vi "Fin_main.vi"(8 "Error In":errorcluster, 11 "Fin Arrangement (SORTED)":u8[](array[numeric])) -> (0 "Error Out":errorcluster)   [LabVIEW 2013]
uses:
  <vilib>/Platform/TimedLoop/XDataNode/timing_clust.ctl
  <vilib>/Platform/TimedLoop/XDataNode/nitl_modes.ctl
  <vilib>/Platform/TimedLoop/XDataNode/wakeup.ctl
  My Computer/Controls/Steering Mode.ctl
  My Computer/Controls/Fin Status.ctl
  <vilib>/platform/TimedLoop/XDataNode/XDataNode.xnode
  <vilib>/Platform/TimedLoop/XDataNode/XDNodeRunTimeDep.lvlib
panel:
  out "x-y":dbl
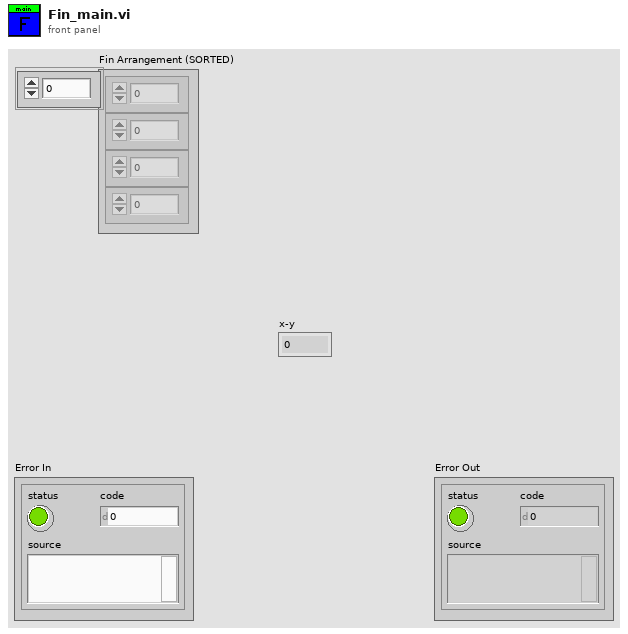
[diagram p1: front panel]
types:
  T1 = typedef "XDNodeRunTimeDep.lvlib/timing_clust.ctl" = cluster{"Expected End [f-1]":u64, "Actual End [f-1]":u64, "Finished Late? [f-1]":bool, "Expected End [i-1]":u64, "Actual End [i-1]":u64, "Finished Late? [i-1]":bool, "Expected Start [i]":u64, "Actual Start [i]":u64, "Expected Start [f]":u64, "Actual Start [f]":u64, "Source Name":string, "Structure Name":string, "Period":i64, "Deadline":i64, "Offset":i64, "Start":i64, "Priority":i32, "Timeout":i32, "Mode":T2, "Wakeup Reason":T3, "Error":errorcluster, "Source Type":string, "Secondary Source Type":string, "Global End Time":u64, "Global Start Time":u64, "Frame Duration":u64, "Iteration Duration":u64, "Assigned CPU":i32, "I/O Scan Engine Mode":u32}
  T2 = typedef "XDNodeRunTimeDep.lvlib/nitl_modes.ctl" = enum32{"No Change", "Process missed periods, maintain original phase", "Discard missed periods, maintain original phase", "Process missed periods, ignore original phase", "Discard missed periods, ignore original phase"}
  T3 = typedef "XDNodeRunTimeDep.lvlib/wakeup.ctl" = enum32{"Normal", "Aborted", "Asynchronous wakeup", "Timing source error", "Timed loop error", "Timeout"}
  T4 = typedef "Steering Mode.ctl" = enum16{"Intuitive Steering", "Control Allocation", "Individually"}
  T5 = typedef "Servo Position.ctl" = dbl[][]
  T6 = typedef "Fin Status.ctl" = u32[]
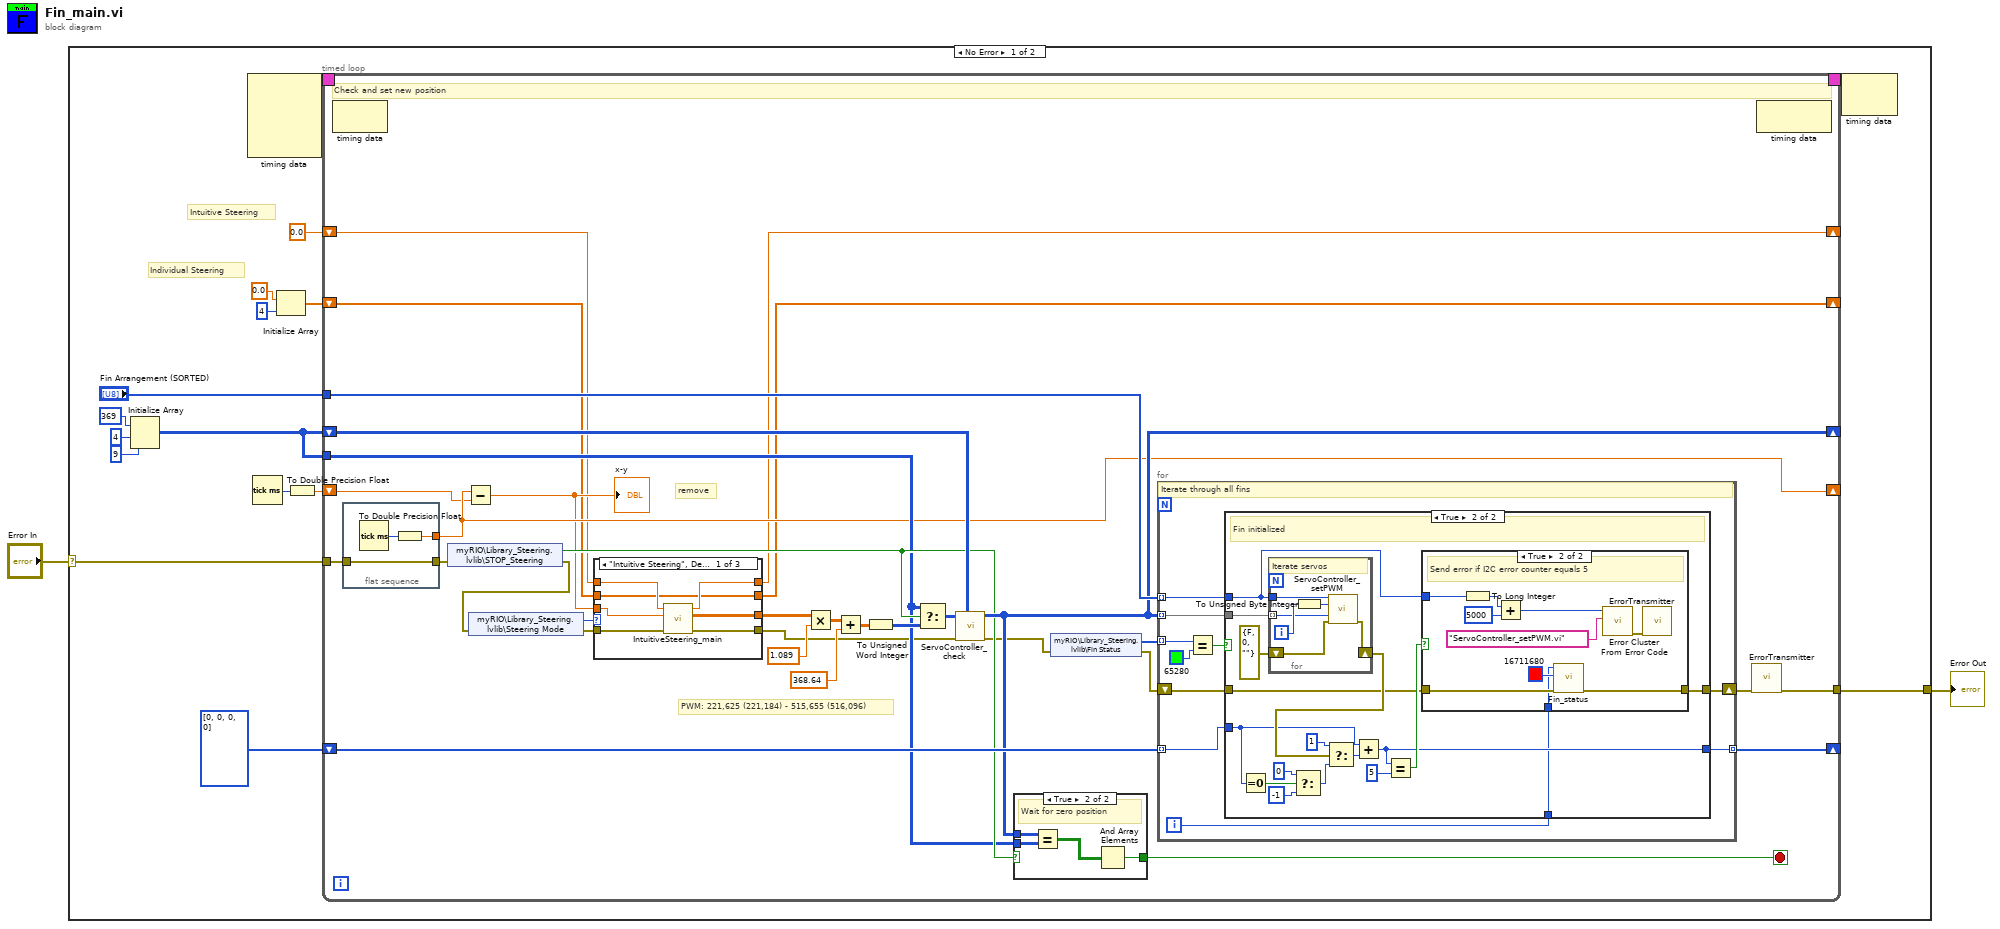
[diagram p0: block diagram]
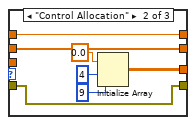
[diagram p2: hidden frame]
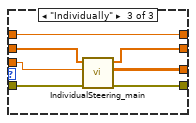
[diagram p3: hidden frame]
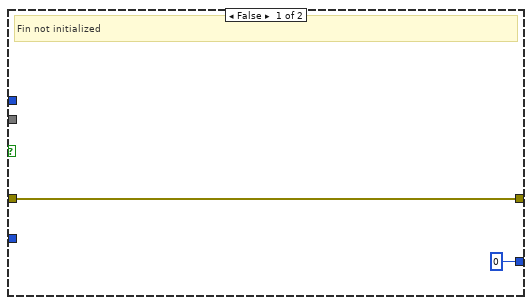
[diagram p5: hidden frame]
diagram:
  n1 = case shown="No Error" "Error In" {
    selector: "Error In" -> [w12 w131]
    tunnel: [w11 w131] -> w1
    frame No Error {
      # "Individual Steering"
      # "Intuitive Steering"
      n2 = Initialize Array(u16 369 ("element"), 4 ("dimension size"), 9 ("dimension size")) -> (w15:u16[][])
      n3 = node-c288() -> (w10:T1)  [unwired: 4 in]
      n4 = Tick Count (ms)() -> (millisecond timer value=w7:u32)
      n5 = Initialize Array(0.0 ("element"), 4 ("dimension size")) -> (w3:dbl[])
      n6 = To Double Precision Float(number=w7) -> (double precision float=w6:dbl)
      n7 = timed-loop {
        tunnel: "Fin Arrangement (SORTED)" -> [w51]
        shift-right: [w42] -> _
        shift-left: w15 -> [w48]
        tunnel: w15 -> [w33]
        shift-right: [w46] -> _
        shift-left: i8[] [0, 0, 0, 0] -> [w47]
        tunnel: w12 -> [w31]
        tunnel: [w38] -> w11
        timing: w10 -> [_]
        timing-out: [_] -> w9
        shift-right: [w22] -> _
        shift-left: 0.0 ("Time In") -> [w23]
        shift-right: [w29] -> _
        shift-left: w6 -> [w28]
        shift-right: [w20] -> _
        shift-left: w3 -> [w19]
        stop <- w40 stop-if-true
        # "remove"
        # "PWM: 221,625 (221,184) - 515,655 (516,096)"
        # "Check and set new position"
        n8 = node-c288() -> ()  [unwired: 1 in, 1 out]
        n9 = flat-sequence {
          tunnel: [w75] -> w30
          tunnel: w31 -> [w75]
          tunnel: [w73] -> w29
          frame #0 {
            n10 = Tick Count (ms)() -> (millisecond timer value=w74:u32)
            n11 = To Double Precision Float(number=w74) -> (double precision float=w73:dbl)
          }
        }
        n12 = shared-variable "myRIO\\Library_Steering.lvlib\\STOP_Steering"(error in=w30) -> (w41:bool, error out=w32:errorcluster)
        n13 = Subtract(x=w29, y=w28) -> (x-y=w24:dbl)
        "x-y" <- w24
        n14 = shared-variable "myRIO\\Library_Steering.lvlib\\Steering Mode"(error in=w32) -> (w27:T4, error out=w26:errorcluster)
        n15 = case shown="\"Intuitive Steering\", Default" w27 {
          tunnel: w26 -> [w58 w65 w72]
          tunnel: [w57 w65 w71] -> w25
          tunnel: w24 -> [w56 _ w67]
          tunnel: w23 -> [w55 w64 w66]
          tunnel: [w54 w64 w66] -> w22
          tunnel: [w53 w59 w70] -> w21
          tunnel: [w52 w63 w69] -> w20
          tunnel: w19 -> [w52 w63 w68]
          frame "Intuitive Steering", Default {
            n16 = call "IntuitiveSteering_main.vi"("Error In"=w58, "dt"=w56, "Time In"=w55) -> ("Error Out"=w57:errorcluster, "Servo Position"=w53:T5, "Time Out"=w54:dbl)  [unwired: 6 in]
          }
          frame "Control Allocation" {
            n17 = Initialize Array(0.0 ("element"), 4 ("dimension size"), 9 ("dimension size")) -> (w59:dbl[][])
          }
          frame "Individually" {
            n18 = call "IndividualSteering_main.vi"("Error In"=w72, "dt"=w67, "Times In"=w68) -> ("Error Out"=w71:errorcluster, "Servo Position"=w70:T5, "Times Out"=w69:dbl[])  [unwired: 6 in]
          }
        }
        n19 = Multiply(x=w21, y=1.089) -> (x*y=w50:T5)
        n20 = Add(x=w50, y=368.64) -> (x+y=w49:T5)
        n21 = To Unsigned Word Integer(number=w49) -> (unsigned 16bit integer=w44:u16[][])
        n22 = Select(t=w33, s=w41, f=w44) -> (s? t:f=w43:u16[][])
        n23 = call "ServoController_check.vi"("Servo Position Old (U16)"=w48, "Error In"=w25, "Servo Position In (U16)"=w43) -> ("Error Out"=w39:errorcluster, "Servo Position Out (U16)"=w42:u16[][])  [unwired: 7 in]
        n24 = case shown="True" w41 {
          selector: w41 -> [w78 _]
          tunnel: w42 -> [_ w80]
          tunnel: [w78 w81] -> w40
          tunnel: w33 -> [_ w79]
          frame False {
            # "Continue"
          }
          frame True {
            # "Wait for zero position"
            n25 = Equal?(x=w80, y=w79) -> (x = y?=w82:bool[][])
            n26 = And Array Elements(Boolean array=w82) -> (logical AND=w81:bool)
          }
        }
        n27 = shared-variable "myRIO\\Library_Steering.lvlib\\Fin Status"(error in=w39) -> (w45:T6, error out=w37:errorcluster)
        n28 = for {
          tunnel: w51 -> [w92] mode=indexing
          tunnel: w42 -> [w91] mode=indexing
          tunnel: w45 -> [w89] mode=indexing
          tunnel: w47 -> [w87] mode=indexing
          tunnel: [w86] -> w46 mode=indexing
          shift-right: [w84] -> w36
          shift-left: w37 -> [w85]
          i -> [w83]
          # "Iterate through all fins"
          n29 = Equal?(x=w89, y=u32 65280 ("Round Color Box")) -> (x = y?=w88:bool)
          n30 = case shown="True" w88 {
            tunnel: w92 -> [_ w99]
            tunnel: w91 -> [_ w111]
            tunnel: w87 -> [_ w104]
            tunnel: [i8 0 w106] -> w86
            tunnel: w85 -> [w93 w97]
            tunnel: [w93 w96] -> w84
            tunnel: w83 -> [_ w95]
            frame False {
              # "Fin not initialized"
            }
            frame True {
              # "Fin initialized"
              n31 = Equal To 0?(x=w104) -> (x = 0?=w101:bool)
              n32 = for {
                tunnel: w99 -> [w128]
                tunnel: w111 -> [w124] mode=indexing
                shift-right: [w125] -> w108
                shift-left: errorcluster {"status"=FALSE, "code"=0, "source"=""} ("error constant") -> [w123]
                i -> [w126]
                # "Iterate servos"
                n33 = To Unsigned Byte Integer(number=w126) -> (unsigned 8bit integer=w127:u8)
                n34 = call "ServoController_setPWM.vi"("Servo Controller Index"=w128, "PWM Channel"=w127, "Off (duty-cycle)"=w124, "Error In"=w123) -> ("Error Out"=w125:errorcluster)  [unwired: 11 in]
              }
              n35 = Select(t=i8 0 ("dimension size"), s=w101, f=i8 -1 ("dimension size")) -> (s? t:f=w100:i8)
              n36 = Select(t=i8 1 ("dimension size"), s=w108, f=w100) -> (s? t:f=w109:i8)
              n37 = Add(x=w104, y=w109) -> (x+y=w106:i8)
              n38 = Equal?(x=w106, y=i8 5) -> (x = y?=w107:bool)
              n39 = case shown="True" w107 {
                tunnel: w99 -> [_ w119]
                tunnel: w97 -> [w112 w115]
                tunnel: [w112 w114] -> w96
                tunnel: w95 -> [_ w113]
                frame False {
                }
                frame True {
                  # "Send error if I2C error counter equals 5"
                  n40 = To Long Integer(number=w119) -> (32bit integer=w117:i32)
                  n41 = Add(x=w117, y=5000 ("code")) -> (x+y=w118:i32)
                  n42 = call "Fin_status.vi"("Error In"=w115, "Round Color Box"=u32 16711680, "Fin Index"=w113) -> ("Error Out"=w114:errorcluster)  [unwired: 8 in]
                  n43 = call <vilib>:"Error Cluster From Error Code.vi"("error message (\"\")"="ServoController_setPWM.vi" ("source"), "error code (0)"=w118) -> ("error out"=w116:errorcluster)  [unwired: 7 in]
                  n44 = call "ErrorTransmitter.vi"("Error In"=w116) -> ()  [unwired: 10 in, 1 out]
                }
              }
            }
          }
        }
        n45 = call "ErrorTransmitter.vi"("Error In"=w36) -> ("Error Out"=w38:errorcluster)  [unwired: 10 in]
        n46 = node-c288() -> ()  [unwired: 1 in, 1 out]
      }
      n47 = node-c288(w9) -> ()  [unwired: 1 out]
    }
    frame Error {
    }
  }
  "Error Out" <- w1
